vi "Driver VISA Clear.vi"(8 "error in (no error)":errorcluster, 9 "Timeout":u32=200, 10 "Read Length":u32=1024, 11 "VISA resource name":refnum<visa-resource-name>) -> (0 "error out":errorcluster, 2 "Receive":string, 3 "VISA resource name out":refnum<visa-resource-name>)   [LabVIEW 2020]
panel:
  out "Length":i32
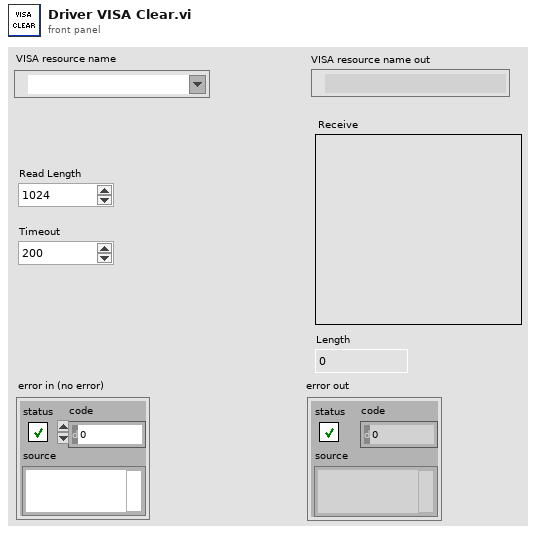
[diagram p1: front panel]
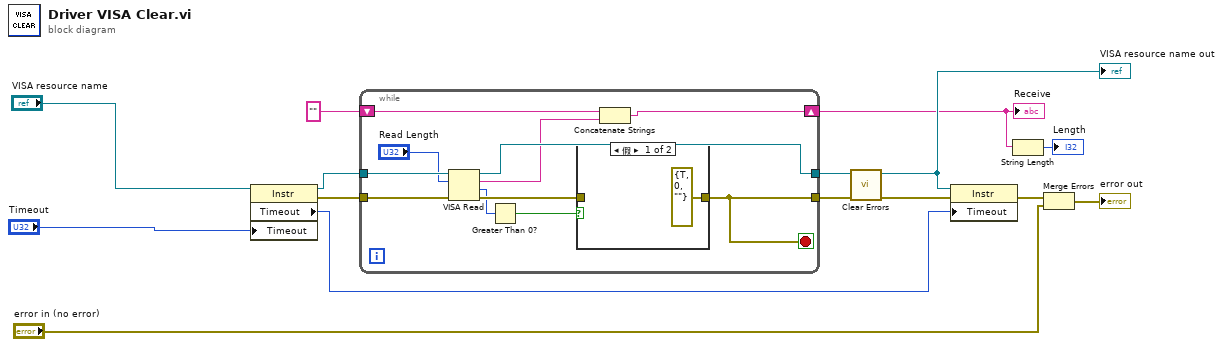
[diagram p0: block diagram]
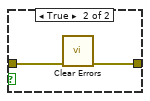
[diagram p2: hidden frame]
diagram:
  n1 = property class="Instr"(reference="VISA resource name", "Timeout"="Timeout") -> (reference out=w7:refnum<visa-resource-name>, error out=w13:errorcluster, "Timeout"=w10:u32)  [unwired: 1 in]
  n2 = while {
    tunnel: w7 -> [w23]
    tunnel: [w24] -> w11
    tunnel: w13 -> [w25]
    tunnel: [w15] -> w9
    shift-right: [w18] -> w3
    shift-left: "" -> [w20]
    stop <- w15 stop-if-true
    n3 = VISA Read(VISA resource name=w23, byte count="Read Length", error in (no error)=w25) -> (VISA resource name out=w24:refnum<visa-resource-name>, read buffer=w19:string, return count=w17:u32, error out=w21:errorcluster)
    n4 = Greater Than 0?(x=w17) -> (x > 0?=w16:bool)
    n5 = case shown="假" w16 {
      tunnel: [errorcluster {"status"=TRUE, "code"=0, "source"=""} ("error out") w28] -> w15
      tunnel: w21 -> [_ w27]
      frame False {
      }
      frame True {
        n6 = call <vilib>:"Clear Errors.vi"("error in (no error)"=w27) -> ("error out"=w28:errorcluster)  [unwired: 5 in, 1 out]
      }
    }
    n7 = Concatenate Strings(w20, w19) -> (w18:string)
  }
  "VISA resource name out" <- w11
  "Receive" <- w3
  n8 = call <vilib>:"Clear Errors.vi"("error in (no error)"=w9) -> ("error out"=w1:errorcluster)  [unwired: 5 in, 1 out]
  n9 = property class="Instr"(reference=w11, error in=w1, "Timeout"=w10) -> (error out=w8:errorcluster)  [unwired: 1 out]
  n10 = String Length(string=w3) -> (length=→"Length":i32)
  n11 = Merge Errors(w8, "error in (no error)") -> (→"error out":errorcluster)
